vi "getThreshold.vi"(8 "error in (no error)":errorcluster, 11 "reference in":refnum<class "subject.lvclass">) -> (0 "error out":errorcluster, 3 "reference out":refnum<class "subject.lvclass">)   [LabVIEW 2015, in "subject.lvclass"]
uses:
  subject.lvclass
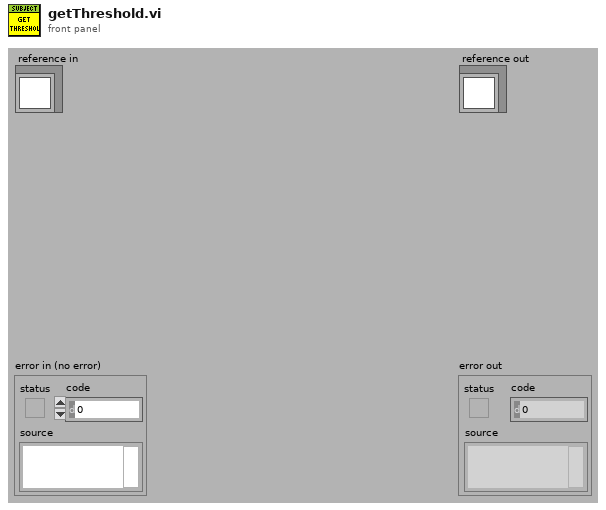
[diagram p1: front panel]
types:
  T1 = typedef "subject.lvclass/ObjectAttributesRef.ctl" = refnum<data-value>
  T2 = typedef "subject.lvclass/ObjectAttributes.ctl" = cluster{"MyAttribute":dbl, "data":cluster{"Ve_warm":dbl[], "time_warm":dbl[], "name":string, "phase":dbl[], "VCO2":dbl[], "VO2":dbl[], "PetCO2":dbl[], "RQ":dbl[], "HR":dbl[], "Ve_warm_inter":dbl[], "time_warm_inter":dbl[], "Ve_exer":dbl[], "time_exer":dbl[], "Ve_exer_inter":dbl[], "time_exer_inter":dbl[], "Ve":dbl[], "time":dbl[]}, "results_5l":cluster{"EOV":bool, "osci_amplitude":dbl[], "osci_width":dbl[], "peak_location":dbl[]}, "results_15percent":cluster{"EOV":bool, "osci_amplitude":dbl[], "osci_width":dbl[], "peak_location":dbl[]}, "supportData":cluster{"peaksAmplitude":dbl[], "iPeaksLocation":dbl[], "valesAmplitude":dbl[], "iValesLocation":dbl[], "threshold":dbl, "width_warm":i32, "meanAmpl_warm":i32, "#_peaks":i32}}
  T3 = cluster{"Ve_warm":dbl[], "time_warm":dbl[], "name":string, "phase":dbl[], "VCO2":dbl[], "VO2":dbl[], "PetCO2":dbl[], "RQ":dbl[], "HR":dbl[], "Ve_warm_inter":dbl[], "time_warm_inter":dbl[], "Ve_exer":dbl[], "time_exer":dbl[], "Ve_exer_inter":dbl[], "time_exer_inter":dbl[], "Ve":dbl[], "time":dbl[]}
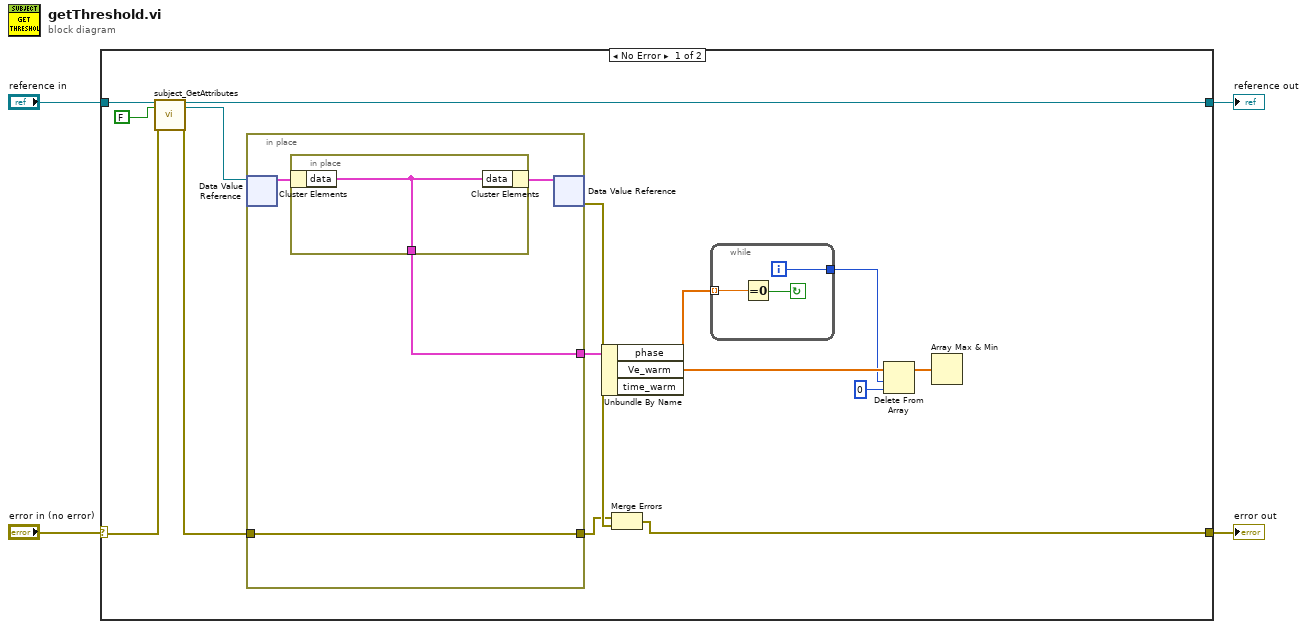
[diagram p0: block diagram]
diagram:
  n1 = case shown="No Error" "error in (no error)" {
    selector: "error in (no error)" -> [w14 w29]
    tunnel: [w19 w29] -> w3
    tunnel: [w12 w28] -> w1
    tunnel: "reference in" -> [w16 w28]
    frame No Error {
      n2 = call "subject_GetAttributes.vi"("reference in"=w16, "return data? (T)"=FALSE, "error in (no error)"=w14) -> ("reference out"=w12:refnum<class "subject.lvclass">, "attributes ref"=w11:T1, "error out"=w13:errorcluster)  [unwired: 13 in, 1 out]
      n3 = in-place {
        in-place-border: w13 -> [w24]
        in-place-border: [w24] -> w17
        in-place-border: [w23] -> w10
        n4 = in-place-dvr #1(w11) -> (w25:T2)  [unwired: 1 out]
        n5 = in-place {
          in-place-border: [w27] -> w23
          n6 = in-place-cluster #2(w25) -> ("data"=w27:T3)
          n7 = in-place-cluster #2("data"=w27) -> (w26:T2)
        }
        n8 = in-place-dvr #1(w26) -> (w18:errorcluster)  [unwired: 1 out]
      }
      n9 = Unbundle By Name(w10) -> ("phase"=w9:dbl[], "Ve_warm"=w8:dbl[])  [unwired: 1 out]
      n10 = Merge Errors(w17, w18) -> (w19:errorcluster)
      n11 = while {
        tunnel: w9 -> [w22] mode=indexing
        tunnel: [w20] -> w7
        i -> [w20]
        stop <- w21 continue-if-true
        n12 = Equal To 0?(x=w22) -> (x = 0?=w21:bool)
      }
      n13 = Delete From Array(array=w8, length=w7, index=0) -> (array with subset deleted=w5:dbl[])  [unwired: 1 out]
      n14 = Array Max & Min(array=w5) -> ()  [unwired: 4 out]
    }
    frame Error {
    }
  }
  "error out" <- w3
  "reference out" <- w1
